vi "h.DETECTION.GetChannelDetectionSettingId.vi"(8 "error in":errorcluster, 10 "Channel Number":u8=1 min=1 max=16, 11 "Connection ID":refnum<k5>) -> (0 "error out":errorcluster, 2 "Detection Setting ID":u8, 3 "Connection ID out":refnum<k5>)   [LabVIEW 2016, in "h.Library.lvlib"]
uses:
  h.Library.lvlib
panel:
  out "Message":string
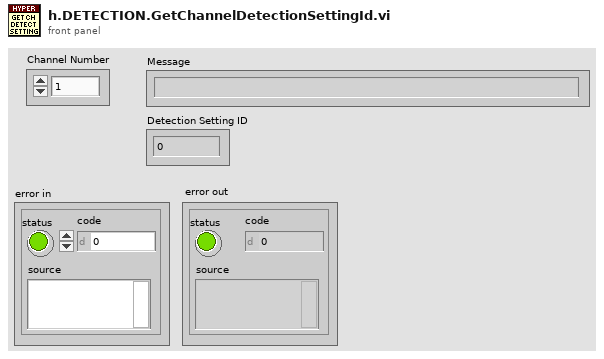
[diagram p1: front panel]
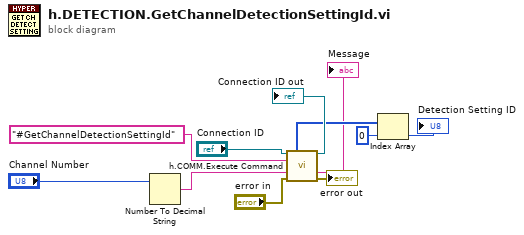
[diagram p0: block diagram]
diagram:
  n1 = Number To Decimal String(number="Channel Number") -> (decimal integer string=w6:string)  [unwired: 1 in]
  n2 = call "h.COMM.Execute Command.vi"("Connection ID"="Connection ID", "Command"="#GetChannelDetectionSettingId", "Argument"=w6, "error in"="error in") -> ("Content"=w4:u8[], "Connection ID out"=→"Connection ID out":refnum<k5>, "Message"=→"Message":string, "error out"=→"error out":errorcluster)  [unwired: 4 in, 4 out]
  n3 = Index Array(array=w4, index=0) -> (element=→"Detection Setting ID":u8)
